vi "AFM_Driver_Manager.Watchdog.vi"(8 "error in (no error)":errorcluster, 11 "AFM_Driver_Manager in":refnum<class "AFM_Driver_Manager.lvclass">) -> (0 "error out":errorcluster, 3 "AFM_Driver_Manager out":refnum<class "AFM_Driver_Manager.lvclass">)   [LabVIEW 2020, in "AFM_Driver_Manager.lvclass"]
uses:
  AFM_Driver_Manager.lvclass
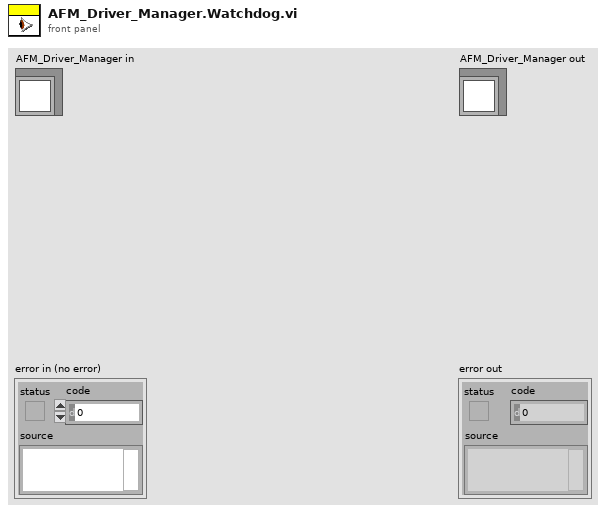
[diagram p1: front panel]
types:
  T1 = typedef "AFM_Driver_Manager.lvclass/AFM_Driver_Manager.PublicEvents.ctl" = cluster{"Lithography Done":refnum<user-event>}
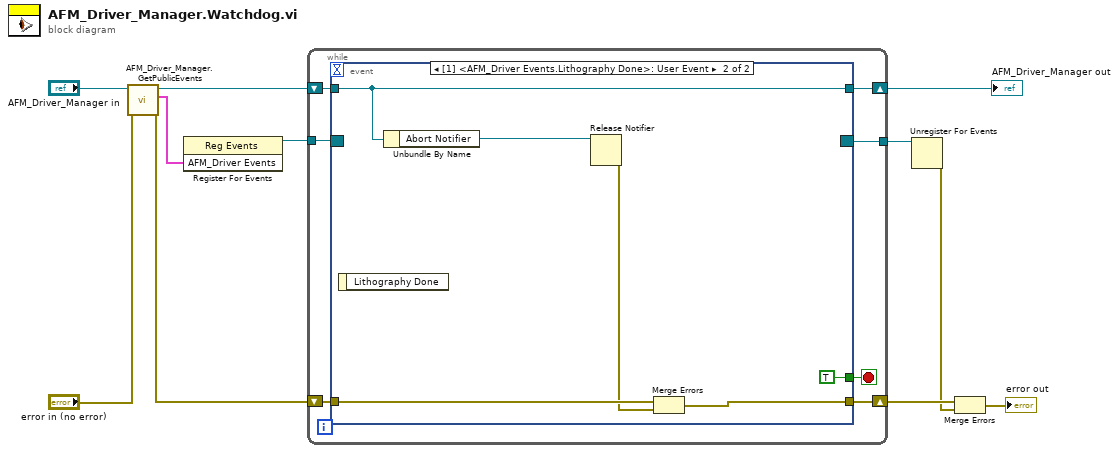
[diagram p0: block diagram]
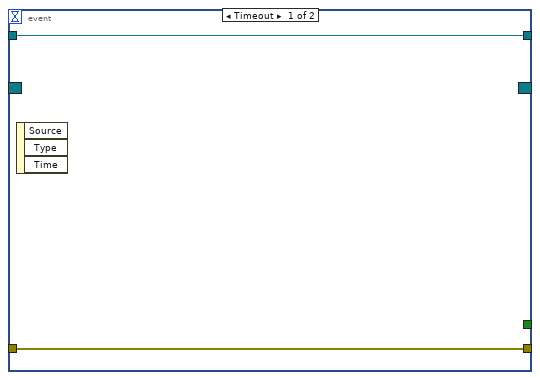
[diagram p2: hidden frame]
diagram:
  n1 = call "AFM_Driver_Manager.GetPublicEvents.vi"("error in (no error)"="error in (no error)", "AFM_Driver_Manager in"="AFM_Driver_Manager in") -> ("error out"=w7:errorcluster, "AFM_Driver Events"=w3:T1, "AFM_Driver_Manager out"=w2:refnum<class "AFM_Driver_Manager.lvclass">)  [unwired: 7 in]
  n2 = register-events(w3) -> (reference out=w11:refnum<event-registration>)  [unwired: 2 in, 1 out]
  n3 = while {
    tunnel: w11 -> [w18]
    tunnel: [w16] -> w8
    shift-right: [w14] -> w6
    shift-left: w7 -> [w15]
    shift-right: [w12] -> w1
    shift-left: w2 -> [w13]
    stop <- w17 stop-if-true
    n4 = event shown="[1] <AFM_Driver Events.Lithography Done>: User Event" {
      selector: w18 -> [_ _]
      dyn-events: [_ _] -> w16
      timeout: _ -> [_ _]
      tunnel: [_ TRUE] -> w17
      tunnel: w15 -> [w20 w23]
      tunnel: [w20 w21] -> w14
      tunnel: w13 -> [w19 w25]
      tunnel: [w19 w25] -> w12
      event Timeout {
        n5 = event-data() -> ()  [unwired: 1 in, 3 out]
      }
      event User Event {
        n6 = event-data() -> ()  [unwired: 1 in, 1 out]
        n7 = Unbundle By Name(w25) -> ("Abort Notifier"=w24:refnum<notifier>)
        n8 = Release Notifier(notifier=w24) -> (error out=w22:errorcluster)  [unwired: 2 in, 2 out]
        n9 = Merge Errors(w23, w22) -> (w21:errorcluster)
      }
    }
  }
  "AFM_Driver_Manager out" <- w1
  n10 = Unregister For Events(event registration refnum=w8) -> (error out=w5:errorcluster)  [unwired: 1 in]
  n11 = Merge Errors(w6, w5) -> (→"error out":errorcluster)
